vi "Implement When VIs.vi"(8 "error in (no error)":errorcluster, 10 "When VIs":path[](array[path]), 11 "Mock Class Generator In":refnum<class "Mock Class Generator.lvclass">) -> (0 "error out":errorcluster, 3 "Mock Class Generator Out":refnum<class "Mock Class Generator.lvclass">)   [LabVIEW 2020, in "Mock Class Generator.lvclass"]
uses:
  Mock Class Generator.lvclass
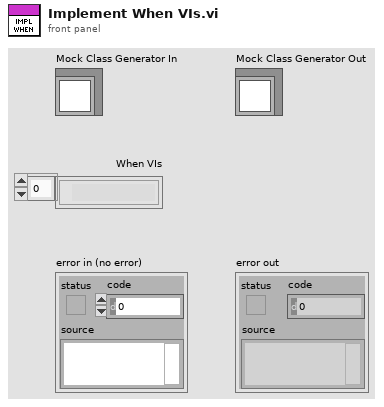
[diagram p1: front panel]
types:
  T1 = enum16{"Invalid Wire Rule", "Required", "Recommended", "Optional", "Dynamic Dispatch"}
  T2 = enum16{"Invalid Wire Rule", "Required", "Recommended", "Optional", "Dynamic Dispatch"}[]
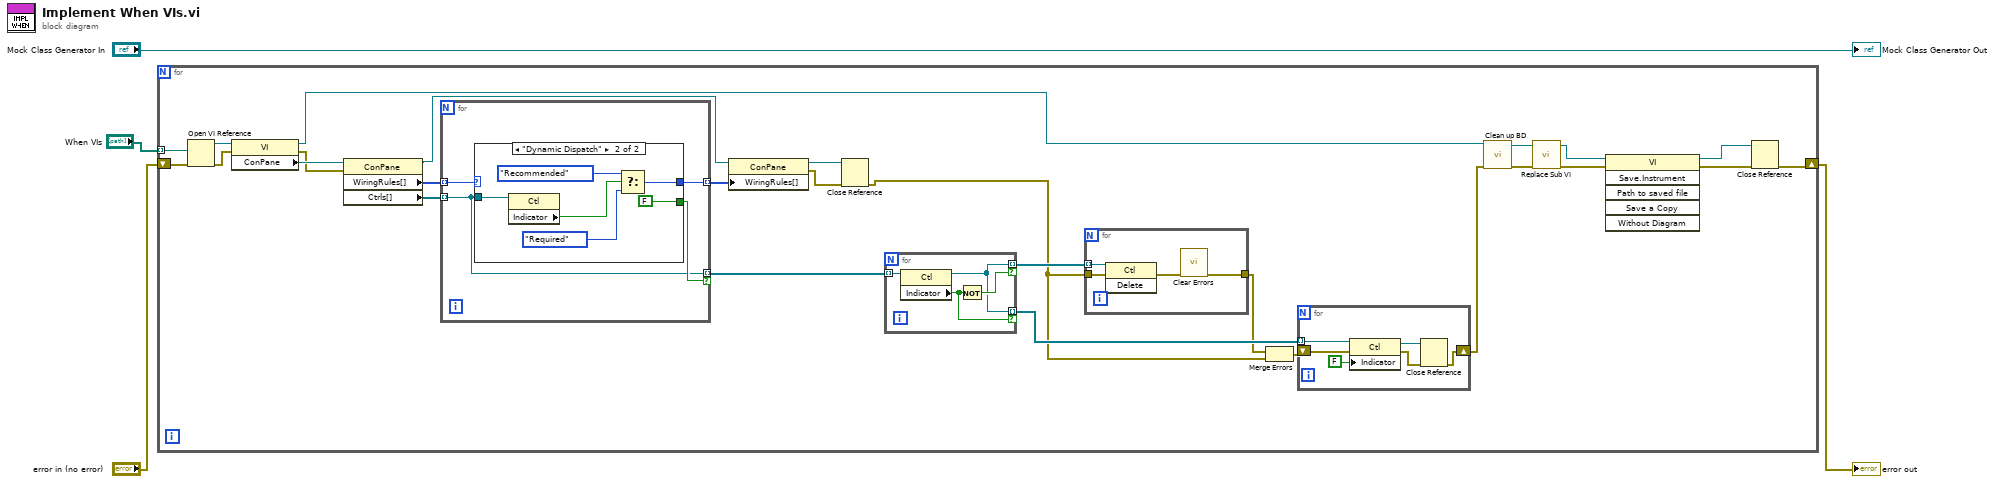
[diagram p0: block diagram]
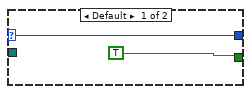
[diagram p2: hidden frame]
diagram:
  n1 = for {
    tunnel: "When VIs" -> [w31] mode=indexing
    shift-right: [w16] -> w1
    shift-left: "error in (no error)" -> [w30]
    n2 = Open VI Reference(vi path=w31, error in (no error)=w30) -> (vi reference=w29:refnum<vi>, error out=w21:errorcluster)  [unwired: 4 in]
    n3 = property class="VI"(reference=w29, error in=w21) -> (reference out=w17:refnum<vi>, error out=w18:errorcluster, "ConPane"=w28:refnum<vi>)
    n4 = property class="ConPane"(reference=w28, error in=w18) -> (reference out=w24:refnum<vi>, "WiringRules[]"=w27:T2, "Ctrls[]"=w25:refnum<vi>[])  [unwired: 1 out]
    n5 = for {
      tunnel: w27 -> [w35] mode=indexing
      tunnel: [w34] -> w26 mode=indexing
      tunnel: w25 -> [w32] mode=indexing
      tunnel: [w32] -> w23 mode=indexing if=w33
      n6 = case shown="\"Dynamic Dispatch\"" w35 {
        selector: w35 -> [w37 _]
        tunnel: [w37 w40] -> w34
        tunnel: [TRUE FALSE] -> w33
        tunnel: w32 -> [_ w41]
        frame Default {
        }
        frame "Dynamic Dispatch" {
          n7 = property class="Ctl"(reference=w41) -> ("Indicator"=w39:bool)  [unwired: 1 in, 2 out]
          n8 = Select(t=T1."Recommended" ("Wire Rule"), s=w39, f=T1."Required" ("Wire Rule")) -> (s? t:f=w40:T1)
        }
      }
    }
    n9 = property class="ConPane"(reference=w24, "WiringRules[]"=w26) -> (reference out=w5:refnum<vi>, error out=w20:errorcluster)  [unwired: 1 in]
    n10 = Close Reference(reference=w5, error in (no error)=w20) -> (error out=w6:errorcluster)
    n11 = for {
      tunnel: [w55] -> w22 mode=indexing if=w56
      tunnel: w23 -> [w57] mode=indexing
      tunnel: [w55] -> w19 mode=indexing if=w54
      n12 = property class="Ctl"(reference=w57) -> (reference out=w55:refnum<vi>, "Indicator"=w54:bool)  [unwired: 1 in, 1 out]
      n13 = Not(x=w54) -> (.not. x?=w56:bool)
    }
    n14 = for {
      tunnel: w22 -> [w53] mode=indexing
      tunnel: w6 -> [w51]
      tunnel: [w50] -> w8
      n15 = invoke class="Ctl" method="Delete"(reference=w53, error in=w51) -> (error out=w52:errorcluster)  [unwired: 1 in, 2 out]
      n16 = call <vilib>:"Clear Errors.vi"("error in (no error)"=w52) -> ("error out"=w50:errorcluster)  [unwired: 5 in, 1 out]
    }
    n17 = Merge Errors(w8, w6) -> (w7:errorcluster)
    n18 = for {
      tunnel: w19 -> [w49] mode=indexing
      shift-right: [w44] -> w14
      shift-left: w7 -> [w45]
      n19 = property class="Ctl"(reference=w49, error in=w45, "Indicator"=FALSE) -> (reference out=w46:refnum<vi>, error out=w47:errorcluster)
      n20 = Close Reference(reference=w46, error in (no error)=w47) -> (error out=w44:errorcluster)
    }
    n21 = call "Clean up BD.vi"("error in (no error)"=w14, "VI in"=w17) -> ("error out"=w15:errorcluster, "VI out"=w12:refnum<vi>)  [unwired: 8 in]
    n22 = call "Replace Sub VI.vi"("error in (no error)"=w15, "VI in"=w12) -> ("error out"=w13:errorcluster, "VI out"=w10:refnum<vi>)  [unwired: 8 in]
    n23 = invoke class="VI" method="Save.Instrument"(reference=w10, error in=w13) -> (reference out=w9:refnum<vi>, error out=w11:errorcluster)  [unwired: 4 in, 4 out]
    n24 = Close Reference(reference=w9, error in (no error)=w11) -> (error out=w16:errorcluster)
  }
  "error out" <- w1
  "Mock Class Generator Out" <- "Mock Class Generator In"
